vi "UPortal List Items.vi"(8 "error in (no error)":errorcluster, 11 ".NET Refnum in":refnum<k24>) -> (0 "error out":errorcluster, 1 "Array":string[](array[string]), 2 "Array 2":string[](array[string]), 3 ".NET Refnum out":refnum<k24>, 5 "Count":i32)   [LabVIEW 2020]
uses:
  System.Windows.Forms
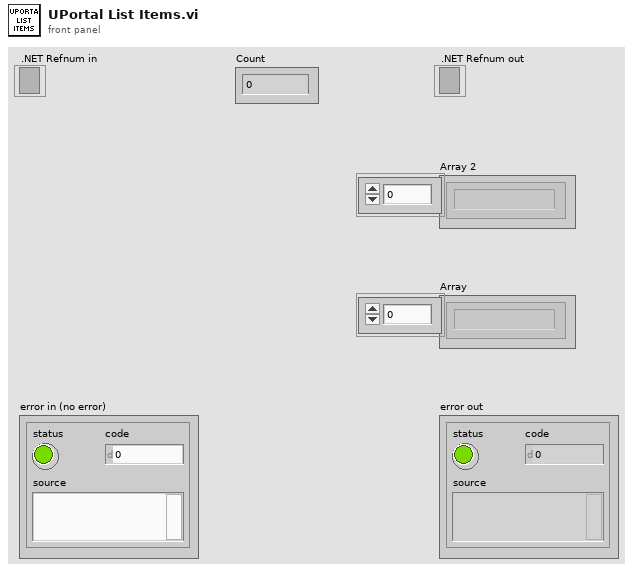
[diagram p1: front panel]
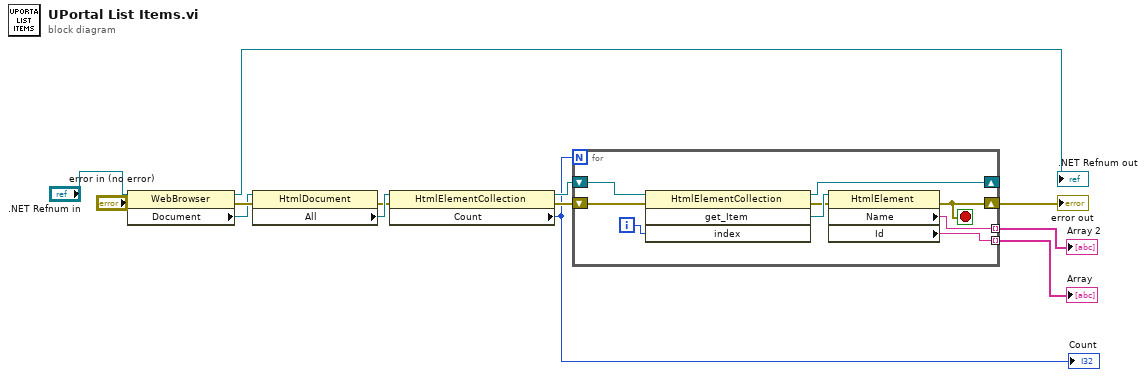
[diagram p0: block diagram]
diagram:
  n1 = property class="WebBrowser"(reference=".NET Refnum in", error in="error in (no error)") -> (reference out=→".NET Refnum out":refnum<k24>, error out=w4:errorcluster, "Document"=w3:refnum<k24>)
  n2 = property class="HtmlDocument"(reference=w3, error in=w4) -> (error out=w2:errorcluster, "All"=w6:refnum<k24>)  [unwired: 1 out]
  n3 = property class="HtmlElementCollection"(reference=w6, error in=w2) -> (reference out=w7:refnum<k24>, error out=w9:errorcluster, "Count"=w5:i32)
  "Count" <- w5
  n4 = for {
    N: w5 -> [_]
    tunnel: [w19] -> w8 mode=indexing
    shift-right: [w16] -> w12
    shift-left: w9 -> [w18]
    tunnel: [w15] -> w10 mode=indexing
    shift-right: [w14] -> _
    shift-left: w7 -> [w22]
    i -> [w21]
    stop <- w16 stop-if-true
    n5 = invoke class="HtmlElementCollection" method="get_Item"(reference=w22, error in=w18, "index"=w21) -> (reference out=w14:refnum<k24>, error out=w17:errorcluster, "get_Item"=w20:refnum<k24>)  [unwired: 1 in, 1 out]
    n6 = property class="HtmlElement"(reference=w20, error in=w17) -> (error out=w16:errorcluster, "Name"=w19:string, "Id"=w15:string)  [unwired: 1 out]
  }
  "error out" <- w12
  "Array" <- w10
  "Array 2" <- w8
